vi "Open VI Not Selected Response.vi"(8 "error in (no error)":errorcluster, 10 "Drive Selection":T1, 11 "Cluster in":refnum<vi>) -> (0 "error out":errorcluster, 3 "References to Items":refnum<vi>[](array[refnum]))   [LabVIEW 2014]
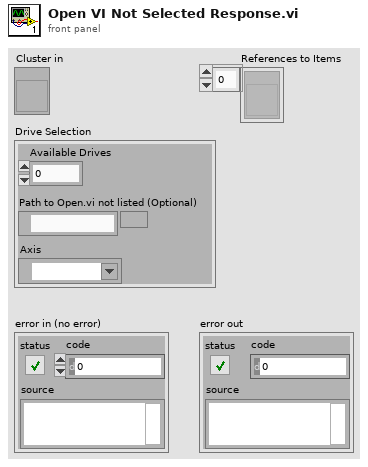
[diagram p1: front panel]
types:
  T1 = cluster{"Available Drives":i32, "Path to Open.vi not listed (Optional)":path, "Axis":refnum<k21>}
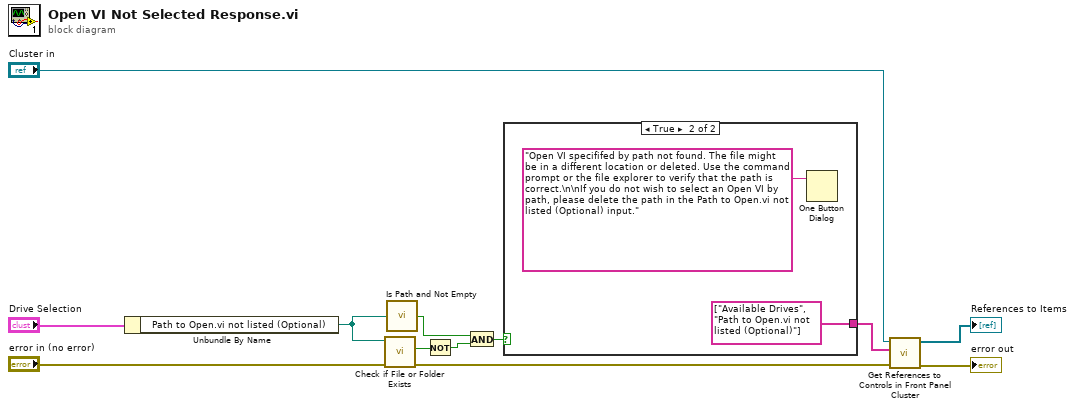
[diagram p0: block diagram]
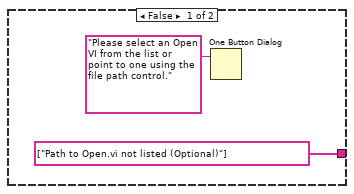
[diagram p2: hidden frame]
diagram:
  n1 = Unbundle By Name("Drive Selection") -> ("Path to Open.vi not listed (Optional)"=w5:path)
  n2 = call <vilib>:"Check if File or Folder Exists.vi"("error in (no error)"="error in (no error)", "path"=w5) -> ("error out"=w7:errorcluster, "file or folder exists?"=w2:bool)  [unwired: 7 in, 1 out]
  n3 = call <vilib>:"Is Path and Not Empty.vi"("path"=w5) -> ("Is Path and Not Empty?"=w3:bool)  [unwired: 4 in]
  n4 = Not(x=w2) -> (.not. x?=w1:bool)
  n5 = And(x=w3, y=w1) -> (x .and. y?=w4:bool)
  n6 = case shown="True" w4 {
    tunnel: [string[] ["Path to Open.vi not listed (Optional)"] string[] ["Available Drives", "Path to Open.vi not listed (Optional)"]] -> w12
    frame False {
      n7 = One Button Dialog(message="Please select an Open VI from the list or point to one using the file path control.") -> ()  [unwired: 1 in, 1 out]
    }
    frame True {
      n8 = One Button Dialog(message="Open VI specififed by path not found. The file might be in a different location or deleted. Use the command prompt or the file explorer to verify that the path is correct.\n\nIf you do not wish to select an Open VI by path, please delete the path in the Path to Open.vi not listed (Optional) input.") -> ()  [unwired: 1 in, 1 out]
    }
  }
  n9 = call "Get References to Controls in Front Panel Cluster.vi"("error in (no error)"=w7, "Items in Cluster"=w12, "Clust Refnum"="Cluster in") -> ("error out"=→"error out":errorcluster, "References to Items"=→"References to Items":refnum<vi>[])  [unwired: 7 in]
